vi "Get Predefined-Page VI.vi"(8 "error in (no error)":errorcluster, 10 "Page":string, 11 "ViewMgr in":refnum<class "ViewMgr.lvclass">) -> (0 "error out":errorcluster, 2 "PageVI Ref":refnum<vi>, 3 "ViewMgr out":refnum<class "ViewMgr.lvclass">)   [LabVIEW 2020, in "CSM-TagDBDisplayContainer.lvlib" / "ViewMgr.lvclass"]
uses:
  ViewMgr.lvclass
  ViewMgr.lvclass/ViewMgr.ctl
  DefaultPage.vi
  CSM-TagDBDisplayContainer.lvlib
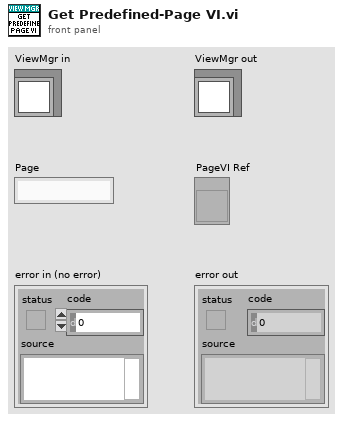
[diagram p1: front panel]
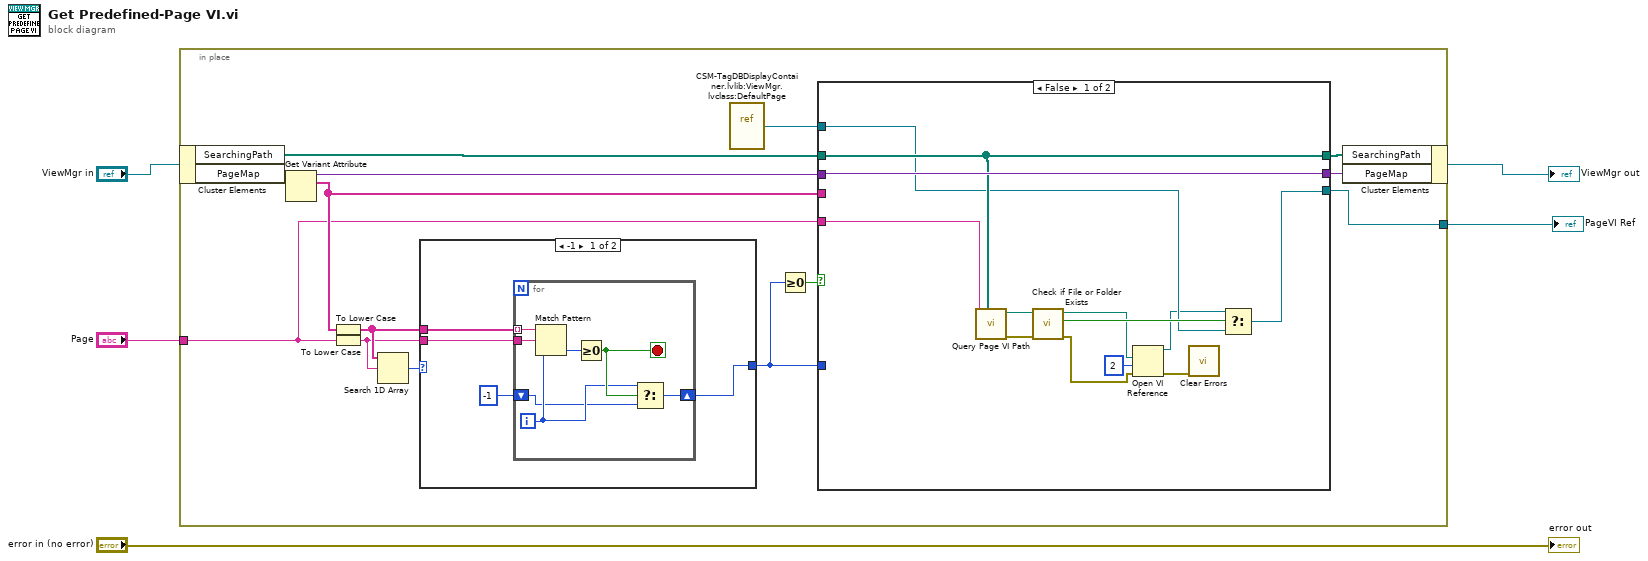
[diagram p0: block diagram]
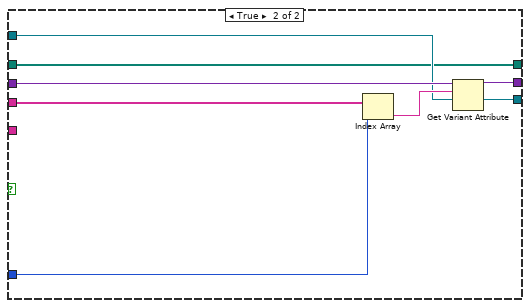
[diagram p2: hidden frame]
diagram:
  n1 = in-place {
    in-place-border: "Page" -> [w8]
    in-place-border: [w12] -> w1
    n2 = in-place-cluster #1("ViewMgr in") -> ("SearchingPath"=w6:path[], "PageMap"=w18:variant)
    n3 = Get Variant Attribute(Variant=w18) -> (duplicate Variant=w17:variant, names=w13:string[])  [unwired: 3 in, 2 out]
    n4 = To Lower Case(string=w13) -> (all lower case string=w15:string[])
    n5 = To Lower Case(string=w8) -> (all lower case string=w14:string)
    n6 = Search 1D Array(1D array=w15, element=w14) -> (index of element=w16:i32)  [unwired: 1 in]
    n7 = case shown="-1" w16 {
      selector: w16 -> [_ w52]
      tunnel: w15 -> [w44 _]
      tunnel: w14 -> [w43 _]
      tunnel: [w41 w52] -> w9
      frame -1 {
        n8 = for {
          tunnel: w44 -> [w49] mode=indexing
          tunnel: w43 -> [w51]
          shift-right: [w45] -> w41
          shift-left: -1 -> [w46]
          i -> [w47]
          stop <- w48 stop-if-true
          n9 = Match Pattern(string=w49, regular expression=w51, offset (0)=w47) -> (offset past match=w50:i32)  [unwired: 3 out]
          n10 = Greater Or Equal To 0?(x=w50) -> (x >= 0?=w48:bool)
          n11 = Select(t=w47, s=w48, f=w46) -> (s? t:f=w45:i32)
        }
      }
      frame Default {
      }
    }
    n12 = vi-ref "CSM-TagDBDisplayContainer.lvlib:ViewMgr.lvclass:DefaultPage.vi"() -> (w11:refnum<vi>)
    n13 = Greater Or Equal To 0?(x=w9) -> (x >= 0?=w10:bool)
    n14 = case shown="False" w10 {
      tunnel: [w32 w40] -> w19
      tunnel: w17 -> [w32 w39]
      tunnel: w9 -> [_ w38]
      tunnel: w13 -> [_ w37]
      tunnel: [w25 w35] -> w12
      tunnel: w11 -> [w26 w34]
      tunnel: w8 -> [w31 _]
      tunnel: [w30 w33] -> w7
      tunnel: w6 -> [w30 w33]
      frame False {
        n15 = call "Query Page VI Path.vi"("searching path"=w30, "page name"=w31) -> ("Error out"=w29:errorcluster, "path"=w28:path)  [unwired: 8 in]
        n16 = call <vilib>:"Check if File or Folder Exists.vi"("error in (no error)"=w29, "path"=w28) -> ("error out"=w21:errorcluster, "file or folder exists?"=w27:bool, "dup path"=w23:path)  [unwired: 7 in]
        n17 = Open VI Reference(vi path=w23, options=2, error in (no error)=w21) -> (vi reference=w22:refnum<vi>, error out=w20:errorcluster)  [unwired: 3 in]
        n18 = call <vilib>:"Clear Errors.vi"("error in (no error)"=w20) -> ()  [unwired: 5 in, 2 out]
        n19 = Select(t=w22, s=w27, f=w26) -> (s? t:f=w25:refnum<vi>)
      }
      frame True {
        n20 = Index Array(array=w37, index=w38) -> (element=w36:string)
        n21 = Get Variant Attribute(Variant=w39, name=w36, default value (empty Variant)=w34) -> (duplicate Variant=w40:variant, value=w35:refnum<vi>)  [unwired: 1 in, 2 out]
      }
    }
    n22 = in-place-cluster #1("SearchingPath"=w7, "PageMap"=w19) -> (→"ViewMgr out":refnum<class "ViewMgr.lvclass">)
  }
  "PageVI Ref" <- w1
  "error out" <- "error in (no error)"
